vi "pregame.vi"() -> ()   [LabVIEW 2025]
uses:
  common/ClientNetworkInterfaceGlobalVariables.vi
  <vilib>/picture/picture.llb/Draw True-Color Pixmap.vi
panel:
  out "Game Field 2":picture
  out "Array 2":string[][](array[string])
  out "which type of box":i32
  out "team number":i32
  out "table of ID&team":i32[][](array[numeric])
  out "Table Control 3":string[][](table) caption="Table Control"
  out "seconds since 1Jan1904 3":timestamp
  out "speed":i32
  out "mountain_density":i32
  out "city_density":i32
  out "width":i32
  out "height":i32
  out "seconds since 1Jan1904 2":timestamp
  out "ACTION":T1
  out "seconds since 1Jan1904":timestamp
  out "map data 2":i32[][](array[numeric])
  in  "stop":bool
  in  "pen":T2={"Width"=1, "Style"=enum."Solid"}
  out "row":dbl
  out "col":dbl
  out "Numeric":i32
  in  "Array":string[][](array[string])
  out "Sent Message 7":string
  in  "Team":u8=1 max=15 step=1
  out "Sent Message 6":string
  out "Sent Message 5":string
  out "Sent Message 4":string
  out "Sent Message 3":string
  out "Sent Message":string
  out "Sent Message 2":string
  in  "Tab Control":enum32{"start", "PreGame", "InGame"}(tab)
  in  "exit":bool
  in  "play":bool
  out "Status":string
  in  "player_name":string
  in  "leave game":bool
  in  "PreGame menu":enum32{"Team", "Options"}(tab)
  in  "spectator":bool caption="Blank Button"
  in  "team5":bool caption="Blank Button"
  in  "team4":bool caption="Blank Button"
  in  "team3":bool caption="Blank Button"
  in  "team2":bool caption="Blank Button"
  in  "team1":bool caption="Blank Button"
  out "Table Control":string[][](table)
  in  "Speed":i32(slide) caption="Slide" scale=1.0..4.0
  in  "Map Width":i32(slide) caption="Slide" scale=10.0..20.0
  in  "Map Height":i32(slide) caption="Slide" scale=10.0..20.0
  in  "City Density":i32(slide) caption="Slide" scale=10.0..40.0
  in  "Mountain Density":i32(slide) caption="Slide" scale=10.0..60.0
  out "Status 2":string
  in  "Ready":bool
  in  "back_to _lobby":bool
  out "Turns":string
  in  "play 2":bool
  out "Game Field":picture
  out "Table Control 2":string[][](table) caption="Table Control"
  # "generals.io"
  # "generals.io"
  # "Protect your general. Capture enemy generals."
  # "Player Name¡G"
  # "Status"
  # "Status"
  # "select your team"
  # "Turn"
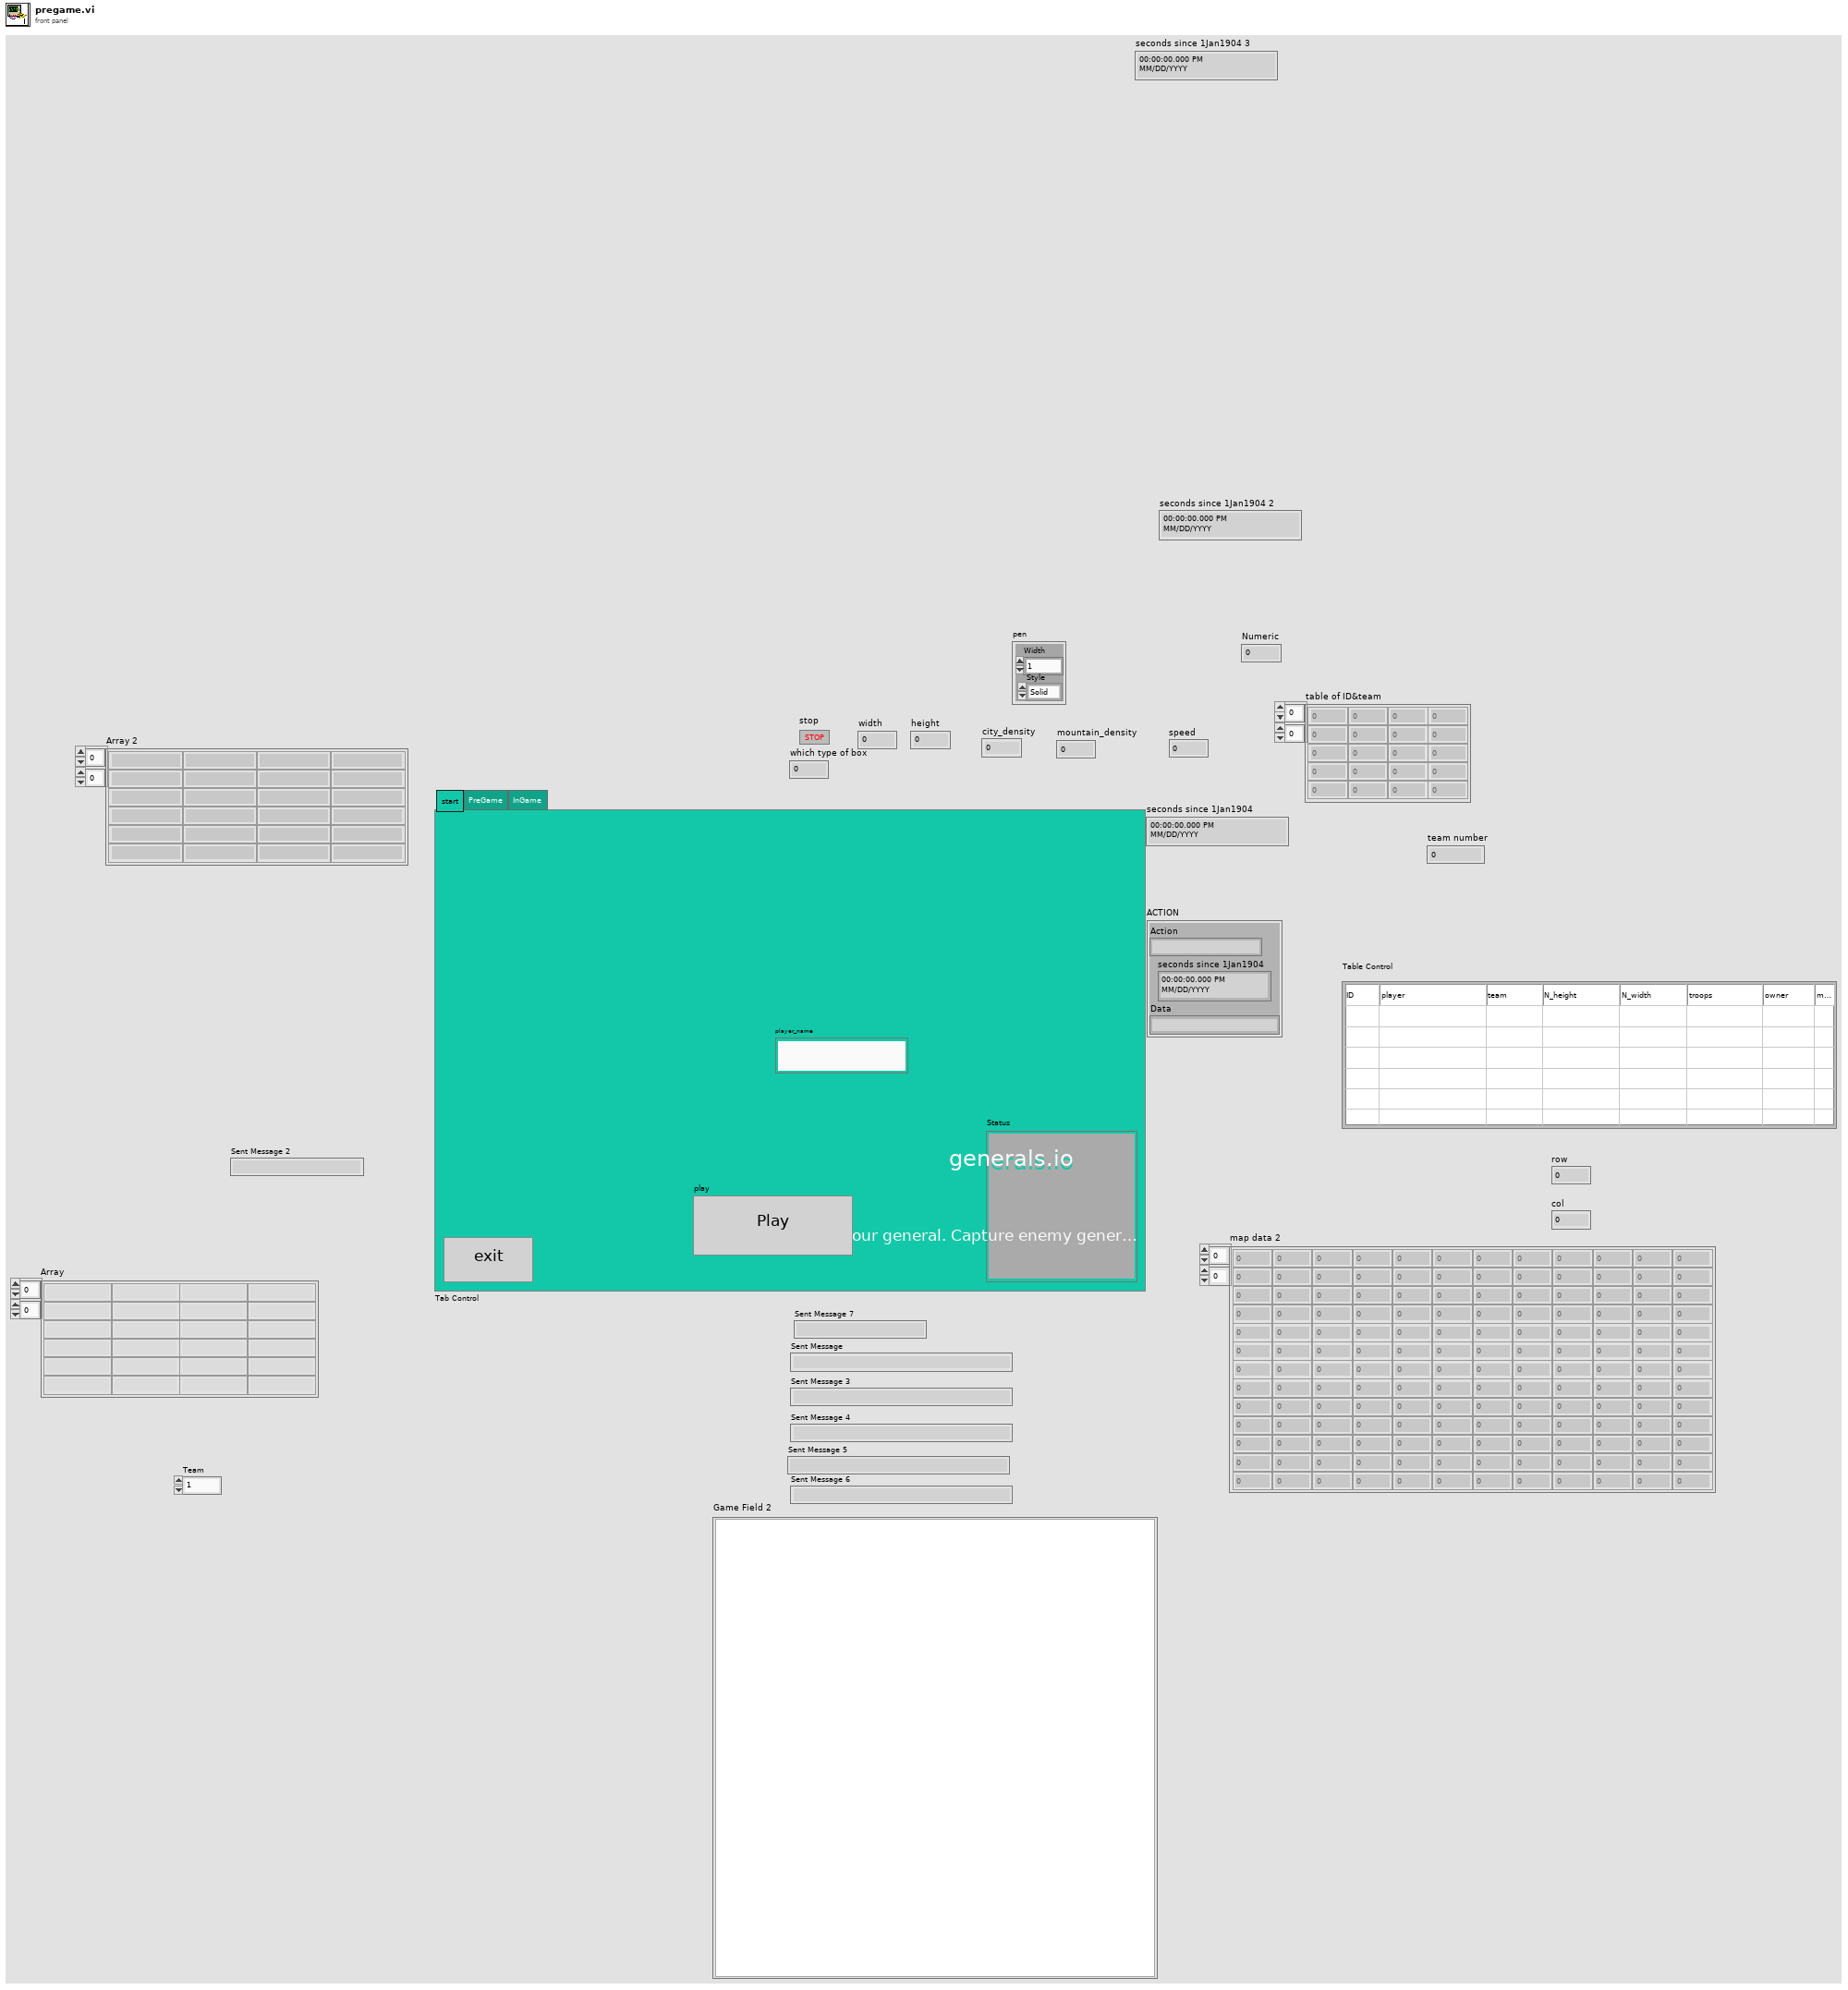
[diagram p1: front panel]
types:
  T1 = cluster{"Action":string, "seconds since 1Jan1904":timestamp, "Data":string}
  T2 = cluster{"Width":i16, "Style":enum32{"Solid", "Dash", "Dot", "DashDot", "DashDotDot"}}
  T3 = cluster{"seconds since 1Jan1904":timestamp, "Data":string}
  T4 = enum16{"Wait Send Queue Ready", "Wait Receive Queue Ready", "Poll Read Queue", "Process Data"}
  T5 = cluster{"Troops":u32, "Owner":i32, "Mountain":bool, "City":bool, "General":bool, "Fog":bool}[]
  T6 = map{u32, cluster{"Name":string, "Team":u8, "Ready":bool, "Host":bool, "Alive":bool, "Color":u32, "Lands":set{cluster{"Row":u32, "Column":u32}}, "Army":u32}}
  T7 = cluster{"Lands":set{cluster{"Row":u32, "Column":u32}}}[]
  T8 = typedef "imagedata.ctl" = cluster{"image type":i32, "image depth":i32, "image":u8[], "mask":u8[], "colors":u32[], "Rectangle":cluster{"left":i16, "top":i16, "right":i16, "bottom":i16}}
  T9 = typedef "LVPoint32TypeDef.ctl" = cluster{"Horizontal":i32, "Vertical":i32}
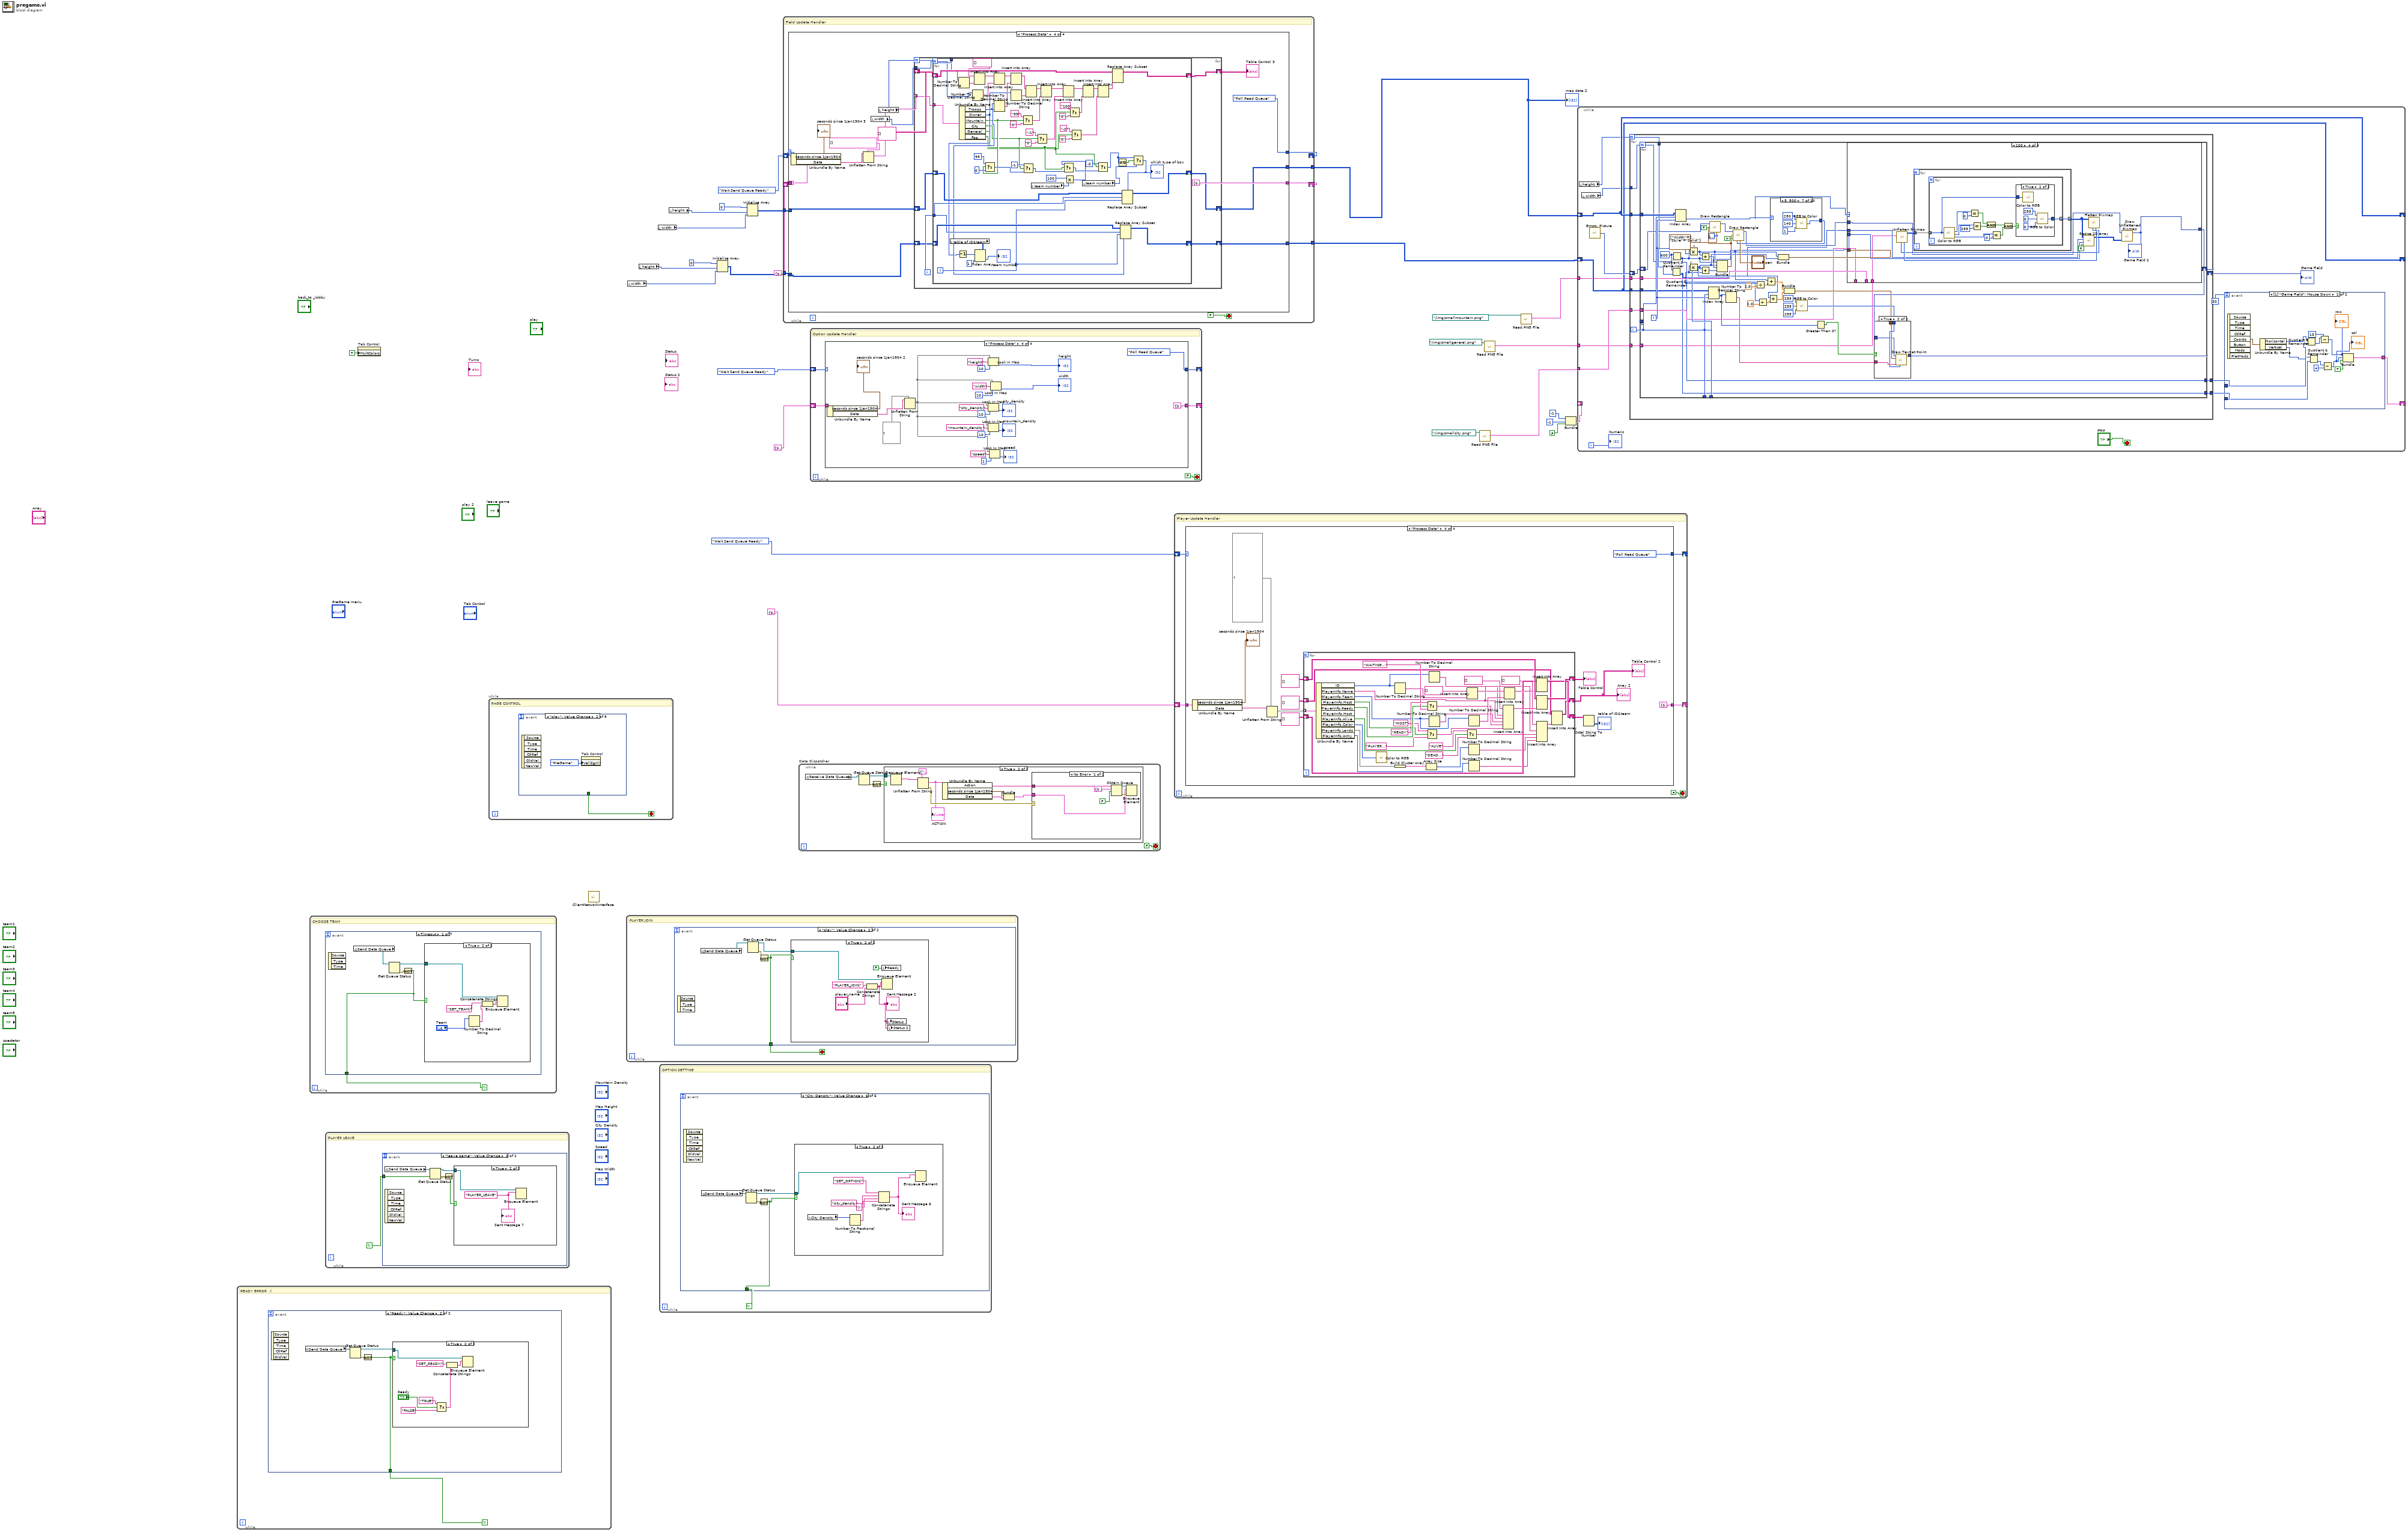
[diagram p0: block diagram]
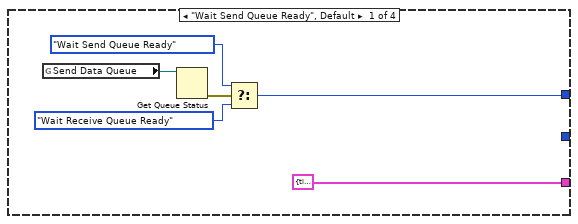
[diagram p2: hidden frame]
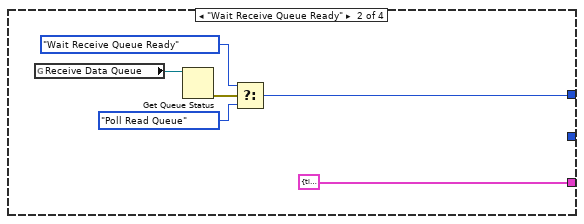
[diagram p3: hidden frame]
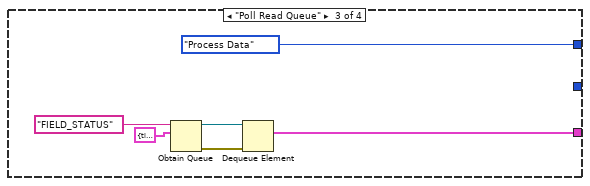
[diagram p4: hidden frame]
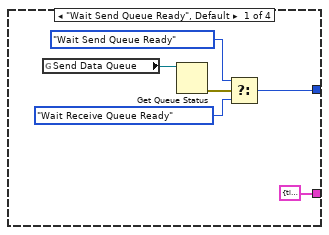
[diagram p5: hidden frame]
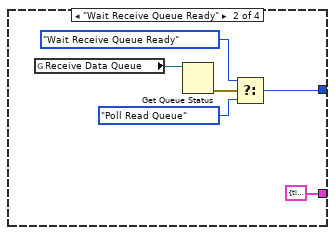
[diagram p6: hidden frame]
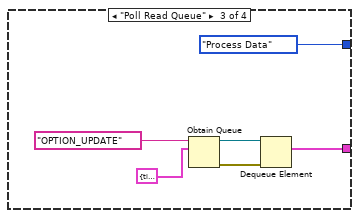
[diagram p7: hidden frame]
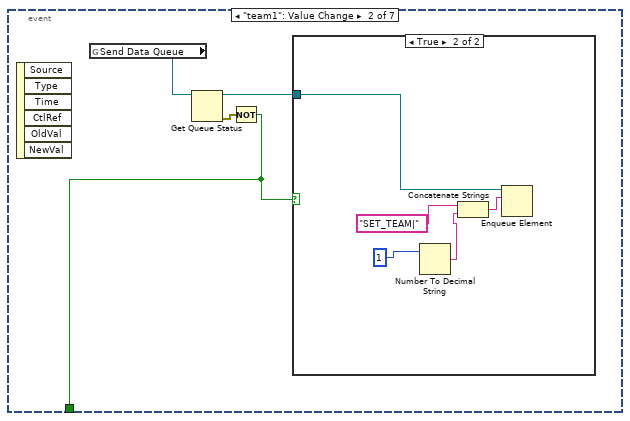
[diagram p9: hidden frame]
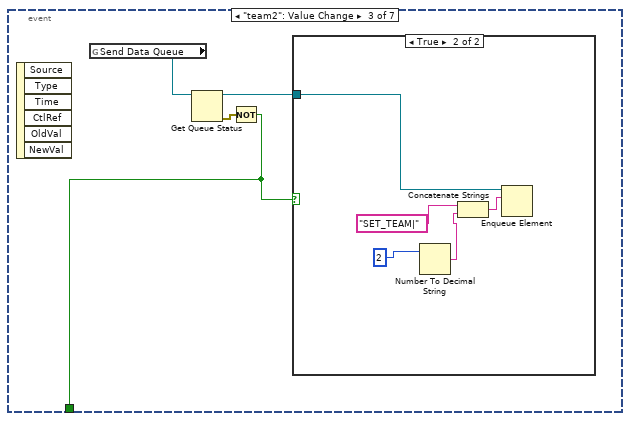
[diagram p11: hidden frame]
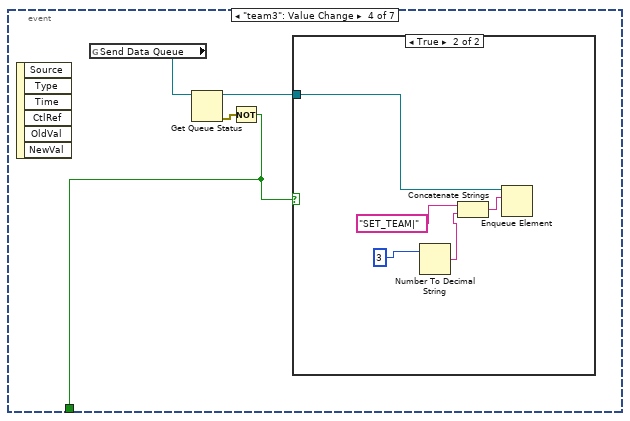
[diagram p13: hidden frame]
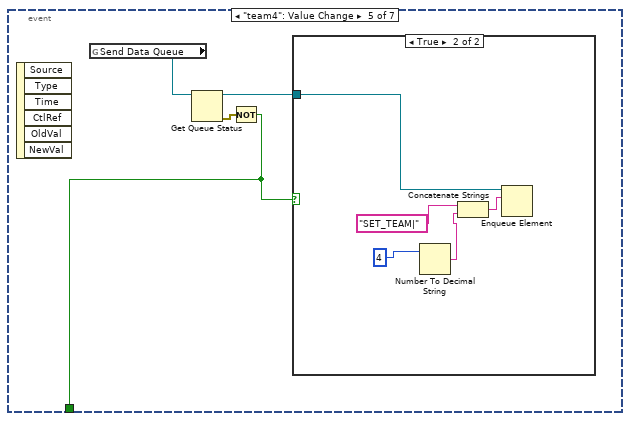
[diagram p15: hidden frame]
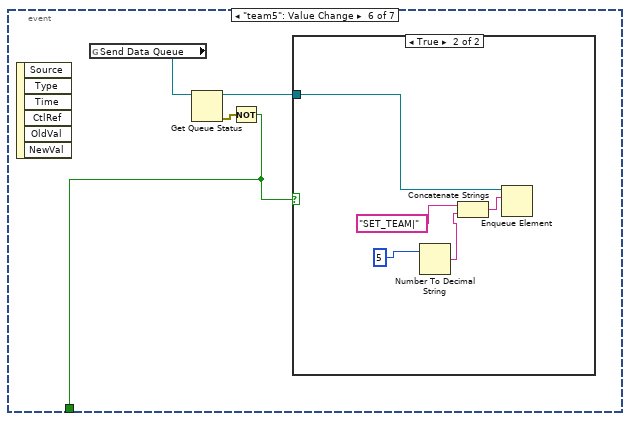
[diagram p17: hidden frame]
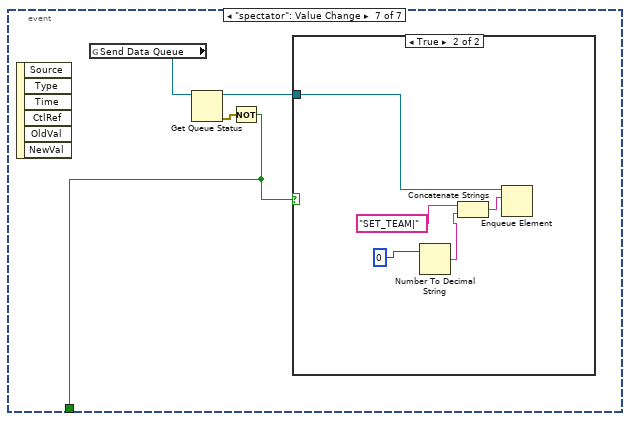
[diagram p19: hidden frame]
diagram:
  n1 = while {
    stop <- w28 continue-if-true
    # "READY ERROR  :("
    n2 = event shown="[1] \"Ready\": Value Change" {
      selector: _ -> [_ _]
      dyn-events: _ -> [_ _]
      timeout: _ -> [_ _]
      tunnel: [_ w29] -> w28
      event Timeout {
        n3 = event-data() -> ()  [unwired: 1 in, 3 out]
      }
      event "Ready": Value Change {
        n4 = event-data() -> ()  [unwired: 1 in, 5 out]
        n5 = global read "ClientNetworkInterfaceGlobalVariables.vi" "Send Data Queue"() -> (w32:refnum<queue>)
        n6 = Get Queue Status(queue=w32) -> (queue out=w31:refnum<queue>, error out=w30:errorcluster)  [unwired: 2 in, 6 out]
        n7 = Not(x=w30) -> (.not. x?=w29:bool)
        n8 = case shown="True" w29 {
          tunnel: w31 -> [_ w37]
          frame False {
          }
          frame True {
            n9 = Select(t="TRUE", s="Ready", f="FALSE") -> (s? t:f=w34:string)
            n10 = Concatenate Strings("SET_READY|" ("string"), w34) -> (w39:string)
            n11 = Enqueue Element(queue=w37, element=w39) -> ()  [unwired: 2 in, 3 out]
          }
        }
      }
    }
  }
  n12 = while {
    stop <- w40 continue-if-true
    # "CHOOSE TEAM"
    n13 = event shown="[0] Timeout" {
      selector: _ -> [_ _ _ _ _ _ _]
      dyn-events: _ -> [_ _ _ _ _ _ _]
      timeout: _ -> [_ _ _ _ _ _ _]
      tunnel: [w42 w51 w60 w69 w78 w87 w96] -> w40
      event Timeout {
        n14 = event-data() -> ()  [unwired: 1 in, 3 out]
        n15 = global read "ClientNetworkInterfaceGlobalVariables.vi" "Send Data Queue"() -> (w44:refnum<queue>)
        n16 = Get Queue Status(queue=w44) -> (queue out=w41:refnum<queue>, error out=w43:errorcluster)  [unwired: 2 in, 6 out]
        n17 = Not(x=w43) -> (.not. x?=w42:bool)
        n18 = case shown="True" w42 {
          tunnel: w41 -> [_ w46]
          frame False {
          }
          frame True {
            n19 = Number To Decimal String(number="Team") -> (decimal integer string=w47:string)  [unwired: 1 in]
            n20 = Concatenate Strings("SET_TEAM|" ("string"), w47) -> (w48:string)
            n21 = Enqueue Element(queue=w46, element=w48) -> ()  [unwired: 2 in, 3 out]
          }
        }
      }
      event "team1": Value Change {
        n22 = event-data() -> ()  [unwired: 1 in, 6 out]
        n23 = global read "ClientNetworkInterfaceGlobalVariables.vi" "Send Data Queue"() -> (w53:refnum<queue>)
        n24 = Get Queue Status(queue=w53) -> (queue out=w50:refnum<queue>, error out=w52:errorcluster)  [unwired: 2 in, 6 out]
        n25 = Not(x=w52) -> (.not. x?=w51:bool)
        n26 = case shown="True" w51 {
          tunnel: w50 -> [_ w55]
          frame False {
          }
          frame True {
            n27 = Number To Decimal String(number=1) -> (decimal integer string=w56:string)  [unwired: 1 in]
            n28 = Concatenate Strings("SET_TEAM|" ("string"), w56) -> (w57:string)
            n29 = Enqueue Element(queue=w55, element=w57) -> ()  [unwired: 2 in, 3 out]
          }
        }
      }
      event "team2": Value Change {
        n30 = event-data() -> ()  [unwired: 1 in, 6 out]
        n31 = global read "ClientNetworkInterfaceGlobalVariables.vi" "Send Data Queue"() -> (w62:refnum<queue>)
        n32 = Get Queue Status(queue=w62) -> (queue out=w59:refnum<queue>, error out=w61:errorcluster)  [unwired: 2 in, 6 out]
        n33 = Not(x=w61) -> (.not. x?=w60:bool)
        n34 = case shown="True" w60 {
          tunnel: w59 -> [_ w64]
          frame False {
          }
          frame True {
            n35 = Number To Decimal String(number=2) -> (decimal integer string=w65:string)  [unwired: 1 in]
            n36 = Concatenate Strings("SET_TEAM|" ("string"), w65) -> (w66:string)
            n37 = Enqueue Element(queue=w64, element=w66) -> ()  [unwired: 2 in, 3 out]
          }
        }
      }
      event "team3": Value Change {
        n38 = event-data() -> ()  [unwired: 1 in, 6 out]
        n39 = global read "ClientNetworkInterfaceGlobalVariables.vi" "Send Data Queue"() -> (w71:refnum<queue>)
        n40 = Get Queue Status(queue=w71) -> (queue out=w68:refnum<queue>, error out=w70:errorcluster)  [unwired: 2 in, 6 out]
        n41 = Not(x=w70) -> (.not. x?=w69:bool)
        n42 = case shown="True" w69 {
          tunnel: w68 -> [_ w73]
          frame False {
          }
          frame True {
            n43 = Number To Decimal String(number=3) -> (decimal integer string=w74:string)  [unwired: 1 in]
            n44 = Concatenate Strings("SET_TEAM|" ("string"), w74) -> (w75:string)
            n45 = Enqueue Element(queue=w73, element=w75) -> ()  [unwired: 2 in, 3 out]
          }
        }
      }
      event "team4": Value Change {
        n46 = event-data() -> ()  [unwired: 1 in, 6 out]
        n47 = global read "ClientNetworkInterfaceGlobalVariables.vi" "Send Data Queue"() -> (w80:refnum<queue>)
        n48 = Get Queue Status(queue=w80) -> (queue out=w77:refnum<queue>, error out=w79:errorcluster)  [unwired: 2 in, 6 out]
        n49 = Not(x=w79) -> (.not. x?=w78:bool)
        n50 = case shown="True" w78 {
          tunnel: w77 -> [_ w82]
          frame False {
          }
          frame True {
            n51 = Number To Decimal String(number=4) -> (decimal integer string=w83:string)  [unwired: 1 in]
            n52 = Concatenate Strings("SET_TEAM|" ("string"), w83) -> (w84:string)
            n53 = Enqueue Element(queue=w82, element=w84) -> ()  [unwired: 2 in, 3 out]
          }
        }
      }
      event "team5": Value Change {
        n54 = event-data() -> ()  [unwired: 1 in, 6 out]
        n55 = global read "ClientNetworkInterfaceGlobalVariables.vi" "Send Data Queue"() -> (w89:refnum<queue>)
        n56 = Get Queue Status(queue=w89) -> (queue out=w86:refnum<queue>, error out=w88:errorcluster)  [unwired: 2 in, 6 out]
        n57 = Not(x=w88) -> (.not. x?=w87:bool)
        n58 = case shown="True" w87 {
          tunnel: w86 -> [_ w91]
          frame False {
          }
          frame True {
            n59 = Number To Decimal String(number=5) -> (decimal integer string=w92:string)  [unwired: 1 in]
            n60 = Concatenate Strings("SET_TEAM|" ("string"), w92) -> (w93:string)
            n61 = Enqueue Element(queue=w91, element=w93) -> ()  [unwired: 2 in, 3 out]
          }
        }
      }
      event "spectator": Value Change {
        n62 = event-data() -> ()  [unwired: 1 in, 6 out]
        n63 = global read "ClientNetworkInterfaceGlobalVariables.vi" "Send Data Queue"() -> (w98:refnum<queue>)
        n64 = Get Queue Status(queue=w98) -> (queue out=w95:refnum<queue>, error out=w97:errorcluster)  [unwired: 2 in, 6 out]
        n65 = Not(x=w97) -> (.not. x?=w96:bool)
        n66 = case shown="True" w96 {
          tunnel: w95 -> [_ w100]
          frame False {
          }
          frame True {
            n67 = Number To Decimal String(number=0) -> (decimal integer string=w101:string)  [unwired: 1 in]
            n68 = Concatenate Strings("SET_TEAM|" ("string"), w101) -> (w102:string)
            n69 = Enqueue Element(queue=w100, element=w102) -> ()  [unwired: 2 in, 3 out]
          }
        }
      }
    }
  }
  n70 = while {
    stop <- w104 continue-if-true
    # "PLAYER LEAVE"
    n71 = event shown="[1] \"leave game\": Value Change" {
      selector: _ -> [_ _]
      dyn-events: _ -> [_ _]
      timeout: _ -> [_ _]
      tunnel: [_ w106] -> w104
      event Timeout {
        n72 = event-data() -> ()  [unwired: 1 in, 3 out]
      }
      event "leave game": Value Change {
        n73 = global read "ClientNetworkInterfaceGlobalVariables.vi" "Send Data Queue"() -> (w107:refnum<queue>)
        n74 = event-data() -> ()  [unwired: 1 in, 6 out]
        n75 = Get Queue Status(queue=w107) -> (queue out=w105:refnum<queue>, error out=w108:errorcluster)  [unwired: 2 in, 6 out]
        n76 = Not(x=w108) -> (.not. x?=w106:bool)
        n77 = case shown="True" w106 {
          tunnel: w105 -> [_ w109]
          frame False {
          }
          frame True {
            w110 = "PLAYER_LEAVE" ("string")
            n78 = Enqueue Element(queue=w109, element=w110) -> ()  [unwired: 2 in, 3 out]
            "Sent Message 7" <- w110
          }
        }
      }
    }
  }
  n79 = property on="Tab Control" class="TabCtl (strict)"("MultColors"=TRUE ("Allow Multiple Colors")) -> ()  [unwired: 2 in, 2 out]
  n80 = while {
    stop <- w111 stop-if-true
    # "PAGE CONTROL"
    n81 = event shown="[1] \"play\": Value Change" {
      selector: _ -> [_ _ _ _ _]
      dyn-events: _ -> [_ _ _ _ _]
      timeout: _ -> [_ _ _ _ _]
      tunnel: [_ _ _ _ "exit"] -> w111
      event Timeout {
        n82 = event-data() -> ()  [unwired: 1 in, 3 out]
      }
      event "play": Value Change {
        n83 = event-data() -> ()  [unwired: 1 in, 6 out]
        n84 = property on="Tab Control" class="TabCtl (strict)"("Val(Sgnl)"=enum32{"start", "PreGame", "InGame"}."PreGame" ("Value (Signaling)")) -> ()  [unwired: 2 in, 2 out]
      }
      event "leave game": Value Change {
        n85 = event-data() -> ()  [unwired: 1 in, 6 out]
        n86 = property on="Tab Control" class="TabCtl (strict)"("Val(Sgnl)"=enum32{"start", "PreGame", "InGame"}."start" ("Value (Signaling)")) -> ()  [unwired: 2 in, 2 out]
      }
      event "back_to _lobby": Value Change {
        n87 = event-data() -> ()  [unwired: 1 in, 6 out]
        n88 = property on="Tab Control" class="TabCtl (strict)"("Val(Sgnl)"=enum32{"start", "PreGame", "InGame"}."PreGame" ("Value (Signaling)")) -> ()  [unwired: 2 in, 2 out]
      }
      event "exit": Value Change {
        n89 = event-data() -> ()  [unwired: 1 in, 6 out]
      }
    }
  }
  n90 = call "ClientNetworkInterface.vi"() -> ()  [unwired: 1 in]
  n91 = while {
    stop <- w116 stop-if-true
    # "PLAYER JOIN"
    n92 = event shown="[1] \"play\": Value Change" {
      selector: _ -> [_ _]
      dyn-events: _ -> [_ _]
      timeout: _ -> [_ _]
      tunnel: [_ w117] -> w116
      event Timeout {
        n93 = event-data() -> ()  [unwired: 1 in, 3 out]
      }
      event "play": Value Change {
        n94 = event-data() -> ()  [unwired: 1 in, 3 out]
        n95 = global read "ClientNetworkInterfaceGlobalVariables.vi" "Send Data Queue"() -> (w118:refnum<queue>)
        n96 = Get Queue Status(queue=w118) -> (queue out=w119:refnum<queue>, error out=w120:errorcluster)  [unwired: 2 in, 6 out]
        n97 = Not(x=w120) -> (.not. x?=w117:bool)
        n98 = case shown="True" w117 {
          tunnel: w119 -> [_ w125]
          frame False {
          }
          frame True {
            n99 = Concatenate Strings("PLAYER_JOIN|" ("string"), "player_name") -> (w122:string)
            "Sent Message 2" <- w122
            n100 = local write "Ready"(FALSE ("Ready")) -> ()
            n101 = Enqueue Element(queue=w125, element=w122) -> ()  [unwired: 2 in, 3 out]
            n102 = local write "Status"(w122) -> ()
            n103 = local write "Status 2"(w122) -> ()
          }
        }
      }
    }
  }
  n104 = local read "width"() -> (w9:i32)
  n105 = local read "height"() -> (w8:i32)
  n106 = local read "width"() -> (w10:i32)
  n107 = while {
    stop <- w126 continue-if-true
    # "OPTION SETTING"
    n108 = event shown="[5] \"City Density\": Value Change" {
      selector: _ -> [_ _ _ _ _ _]
      dyn-events: _ -> [_ _ _ _ _ _]
      timeout: _ -> [_ _ _ _ _ _]
      tunnel: [_ w127 w139 w149 w160 w172] -> w126
      event Timeout {
        n109 = event-data() -> ()  [unwired: 1 in, 3 out]
      }
      event "Map Width": Value Change {
        n110 = event-data() -> ()  [unwired: 1 in, 6 out]
        n111 = global read "ClientNetworkInterfaceGlobalVariables.vi" "Send Data Queue"() -> (w129:refnum<queue>)
        n112 = Get Queue Status(queue=w129) -> (queue out=w128:refnum<queue>, error out=w130:errorcluster)  [unwired: 2 in, 6 out]
        n113 = Not(x=w130) -> (.not. x?=w127:bool)
        n114 = case shown="True" w127 {
          tunnel: w128 -> [_ w131]
          frame False {
          }
          frame True {
            n115 = local read "Map Width"() -> (w132:i32)
            n116 = Number To Fractional String(number=w132) -> (F-format string=w137:string)  [unwired: 3 in]
            n117 = Concatenate Strings("SET_OPTION|" ("string"), "width" ("Option"), "|" ("string"), w137) -> (w133:string)
            "Sent Message" <- w133
            n118 = Enqueue Element(queue=w131, element=w133) -> ()  [unwired: 2 in, 3 out]
          }
        }
      }
      event "Map Height": Value Change {
        n119 = event-data() -> ()  [unwired: 1 in, 6 out]
        n120 = global read "ClientNetworkInterfaceGlobalVariables.vi" "Send Data Queue"() -> (w140:refnum<queue>)
        n121 = Get Queue Status(queue=w140) -> (queue out=w138:refnum<queue>, error out=w141:errorcluster)  [unwired: 2 in, 6 out]
        n122 = Not(x=w141) -> (.not. x?=w139:bool)
        n123 = case shown="True" w139 {
          tunnel: w138 -> [_ w142]
          frame False {
          }
          frame True {
            n124 = local read "Map Height"() -> (w143:i32)
            n125 = Number To Fractional String(number=w143) -> (F-format string=w148:string)  [unwired: 3 in]
            n126 = Concatenate Strings("SET_OPTION|" ("string"), "height" ("Option"), "|" ("string"), w148) -> (w144:string)
            "Sent Message 3" <- w144
            n127 = Enqueue Element(queue=w142, element=w144) -> ()  [unwired: 2 in, 3 out]
          }
        }
      }
      event "Speed": Value Change {
        n128 = event-data() -> ()  [unwired: 1 in, 6 out]
        n129 = global read "ClientNetworkInterfaceGlobalVariables.vi" "Send Data Queue"() -> (w151:refnum<queue>)
        n130 = Get Queue Status(queue=w151) -> (queue out=w150:refnum<queue>, error out=w152:errorcluster)  [unwired: 2 in, 6 out]
        n131 = Not(x=w152) -> (.not. x?=w149:bool)
        n132 = case shown="True" w149 {
          tunnel: w150 -> [_ w153]
          frame False {
          }
          frame True {
            n133 = local read "Speed"() -> (w154:i32)
            n134 = Number To Fractional String(number=w154) -> (F-format string=w159:string)  [unwired: 3 in]
            n135 = Concatenate Strings("SET_OPTION|" ("string"), "speed" ("Option"), "|" ("string"), w159) -> (w155:string)
            "Sent Message 4" <- w155
            n136 = Enqueue Element(queue=w153, element=w155) -> ()  [unwired: 2 in, 3 out]
          }
        }
      }
      event "Mountain Density": Value Change {
        n137 = event-data() -> ()  [unwired: 1 in, 6 out]
        n138 = global read "ClientNetworkInterfaceGlobalVariables.vi" "Send Data Queue"() -> (w162:refnum<queue>)
        n139 = Get Queue Status(queue=w162) -> (queue out=w161:refnum<queue>, error out=w163:errorcluster)  [unwired: 2 in, 6 out]
        n140 = Not(x=w163) -> (.not. x?=w160:bool)
        n141 = case shown="True" w160 {
          tunnel: w161 -> [_ w164]
          frame False {
          }
          frame True {
            n142 = local read "Mountain Density"() -> (w165:i32)
            n143 = Number To Fractional String(number=w165) -> (F-format string=w170:string)  [unwired: 3 in]
            n144 = Concatenate Strings("SET_OPTION|" ("string"), "mountain_density" ("Option"), "|" ("string"), w170) -> (w166:string)
            "Sent Message 5" <- w166
            n145 = Enqueue Element(queue=w164, element=w166) -> ()  [unwired: 2 in, 3 out]
          }
        }
      }
      event "City Density": Value Change {
        n146 = event-data() -> ()  [unwired: 1 in, 6 out]
        n147 = global read "ClientNetworkInterfaceGlobalVariables.vi" "Send Data Queue"() -> (w173:refnum<queue>)
        n148 = Get Queue Status(queue=w173) -> (queue out=w171:refnum<queue>, error out=w174:errorcluster)  [unwired: 2 in, 6 out]
        n149 = Not(x=w174) -> (.not. x?=w172:bool)
        n150 = case shown="True" w172 {
          tunnel: w171 -> [_ w175]
          frame False {
          }
          frame True {
            n151 = local read "City Density"() -> (w176:i32)
            n152 = Number To Fractional String(number=w176) -> (F-format string=w181:string)  [unwired: 3 in]
            n153 = Concatenate Strings("SET_OPTION|" ("string"), "city_density" ("Option"), "|" ("string"), w181) -> (w177:string)
            "Sent Message 6" <- w177
            n154 = Enqueue Element(queue=w175, element=w177) -> ()  [unwired: 2 in, 3 out]
          }
        }
      }
    }
  }
  n155 = local read "height"() -> (w11:i32)
  n156 = Initialize Array(0, w8, w9) -> (w6:i32[][])
  n157 = Initialize Array(0, w11, w10) -> (w4:i32[][])
  n158 = while {
    shift-right: [w189] -> _
    shift-left: T4."Wait Send Queue Ready" -> [w186]
    shift-right: [w187] -> _
    shift-left: T3 {"seconds since 1Jan1904"=timestamp(0 s since 1904-01-01), "Data"=""} ("ActionDataCluster") -> [w188]
    tunnel: w6 -> [w185]
    tunnel: [w184] -> w5
    tunnel: w4 -> [w183]
    tunnel: [w182] -> w3
    stop <- FALSE stop-if-true
    # "Field Update Handler"
    n159 = case shown="\"Process Data\"" w186 {
      tunnel: [w195 w199 T4."Process Data" T4."Poll Read Queue"] -> w189
      tunnel: [T3 {"seconds since 1Jan1904"=timestamp(0 s since 1904-01-01), "Data"=""} ("ActionDataCluster") T3 {"seconds since 1Jan1904"=timestamp(0 s since 1904-01-01), "Data"=""} ("ActionDataCluster") w204 T3 {"seconds since 1Jan1904"=timestamp(0 s since 1904-01-01), "Data"=""} ("ActionDataCluster")] -> w187
      tunnel: w188 -> [_ _ _ w220]
      tunnel: w185 -> [_ _ _ w212]
      tunnel: [_ _ _ w211] -> w184
      tunnel: w183 -> [_ _ _ w210]
      tunnel: [_ _ _ w209] -> w182
      frame "Wait Send Queue Ready", Default {
        n160 = global read "ClientNetworkInterfaceGlobalVariables.vi" "Send Data Queue"() -> (w192:refnum<queue>)
        n161 = Get Queue Status(queue=w192) -> (error out=w196:errorcluster)  [unwired: 2 in, 7 out]
        n162 = Select(t=T4."Wait Send Queue Ready", s=w196, f=T4."Wait Receive Queue Ready") -> (s? t:f=w195:T4)
      }
      frame "Wait Receive Queue Ready" {
        n163 = global read "ClientNetworkInterfaceGlobalVariables.vi" "Receive Data Queue"() -> (w198:refnum<queue>)
        n164 = Get Queue Status(queue=w198) -> (error out=w202:errorcluster)  [unwired: 2 in, 7 out]
        n165 = Select(t=T4."Wait Receive Queue Ready", s=w202, f=T4."Poll Read Queue") -> (s? t:f=w199:T4)
      }
      frame "Poll Read Queue" {
        n166 = Obtain Queue(name (unnamed)="FIELD_STATUS", element data type=T3 {"seconds since 1Jan1904"=timestamp(0 s since 1904-01-01), "Data"=""} ("ActionDataCluster")) -> (queue out=w207:refnum<queue>, error out=w205:errorcluster)  [unwired: 3 in, 1 out]
        n167 = Dequeue Element(queue=w207, error in (no error)=w205) -> (element=w204:T3)  [unwired: 1 in, 3 out]
      }
      frame "Process Data" {
        n168 = Unbundle By Name(w220) -> ("seconds since 1Jan1904"=→"seconds since 1Jan1904 3":timestamp, "Data"=w219:string)
        n169 = Unflatten From String(type=T5 [] ("FieldArray"), binary string=w219) -> (value=w218:T5)  [unwired: 3 in, 2 out]
        n170 = local read "width"() -> (w214:i32)
        n171 = local read "height"() -> (w215:i32)
        n172 = for {
          N: w215 -> [w230]
          shift-right: [w231] -> w213
          shift-left: string[][] [] -> [w232]
          tunnel: w218 -> [w233] mode=indexing
          tunnel: w214 -> [w229]
          shift-right: [w226] -> w209
          shift-left: w210 -> [w227]
          shift-right: [w224] -> w211
          shift-left: w212 -> [w225]
          i -> [w228]
          n173 = for {
            N: w229 -> [w269]
            tunnel: w233 -> [w293]
            shift-right: [w291] -> w231
            shift-left: w232 -> [w292]
            tunnel: w230 -> [w268]
            tunnel: w228 -> [w258]
            shift-right: [w262] -> w226
            shift-left: w227 -> [w263]
            shift-right: [w260] -> w224
            shift-left: w225 -> [w261]
            i -> [w259]
            n174 = local read "table of ID&team"() -> (w256:i32[][])
            n175 = Number To Decimal String(number=w268) -> (decimal integer string=w274:string)  [unwired: 1 in]
            n176 = Unbundle By Name(w293) -> ("Troops"=w257:u32, "Owner"=w252:i32, "Mountain"=w244:bool, "City"=w243:bool, "General"=w242:bool, "Fog"=w241:bool)
            n177 = Decrement(x=w252) -> (x-1=w253:i32)
            n178 = Number To Decimal String(number=w269) -> (decimal integer string=w273:string)  [unwired: 1 in]
            n179 = Insert Into Array(array=string[] [], new element=w274) -> (w271:string[])  [unwired: 1 in]
            n180 = Index Array(array=w256, index (row)=w253, index (col)=1 ("disabled index (col)")) -> (element=→"team number":i32)
            n181 = Select(t=99, s=w244, f=0) -> (s? t:f=w248:i32)
            n182 = Insert Into Array(array=w271, new element=w273) -> (w270:string[])  [unwired: 1 in]
            n183 = Number To Decimal String(number=w257) -> (decimal integer string=w290:string)  [unwired: 1 in]
            n184 = Insert Into Array(array=w270, new element=w290) -> (w289:string[])  [unwired: 1 in]
            n185 = Number To Decimal String(number=w252) -> (decimal integer string=w288:string)  [unwired: 1 in]
            n186 = Select(t="99", s=w244, f="0") -> (s? t:f=w267:string)
            n187 = Select(t=-1, s=w243, f=w248) -> (s? t:f=w247:i32)
            n188 = Insert Into Array(array=w289, new element=w288) -> (w287:string[])  [unwired: 1 in]
            n189 = local read "team number"() -> (w240:i32)
            n190 = Select(t="-1", s=w243, f="0") -> (s? t:f=w266:string)
            n191 = Insert Into Array(array=w287, new element=w267) -> (w286:string[])  [unwired: 1 in]
            n192 = Insert Into Array(array=w286, new element=w266) -> (w285:string[])  [unwired: 1 in]
            n193 = Multiply(x=100 ("t"), y=w240) -> (x*y=w238:i32)
            n194 = Select(t=w238, s=w242, f=w247) -> (s? t:f=w245:i32)
            n195 = Select(t="100", s=w242, f="0") -> (s? t:f=w265:string)
            n196 = Select(t="-2", s=w241, f="0") -> (s? t:f=w264:string)
            n197 = local read "team number"() -> (w235:i32)
            n198 = Insert Into Array(array=w285, new element=w265) -> (w284:string[])  [unwired: 1 in]
            n199 = Select(t=-2, s=w241, f=w245) -> (s? t:f=w236:i32)
            n200 = Insert Into Array(array=w284, new element=w264) -> (w275:string[])  [unwired: 1 in]
            n201 = Replace Array Subset(array=w292, new element=w275) -> (w291:string[][])  [unwired: 2 in]
            n202 = Not Equal To 0?(x=w236) -> (x != 0?=w237:bool)
            n203 = Replace Array Subset(array=w261, new element=w257, index (row)=w258, index (col)=w259) -> (w260:i32[][])
            n204 = Select(t=w236, s=w237, f=w235) -> (s? t:f=w234:i32)
            "which type of box" <- w234
            n205 = Replace Array Subset(array=w263, new element=w234, index (row)=w258, index (col)=w259) -> (w262:i32[][])
          }
        }
        "Table Control 3" <- w213
      }
    }
  }
  "map data 2" <- w3
  n206 = while "Data Dispatcher" {
    stop <- FALSE stop-if-true
    n207 = global read "ClientNetworkInterfaceGlobalVariables.vi" "Receive Data Queue"() -> (w294:refnum<queue>)
    n208 = Get Queue Status(queue=w294) -> (queue out=w295:refnum<queue>, error out=w297:errorcluster)  [unwired: 2 in, 6 out]
    n209 = Not(x=w297) -> (.not. x?=w296:bool)
    n210 = case shown="True" w296 {
      tunnel: w295 -> [_ w307]
      frame False {
      }
      frame True {
        n211 = Dequeue Element(queue=w307) -> (element=w306:string)  [unwired: 2 in, 3 out]
        n212 = Unflatten From String(type=T1 {"Action"="", "seconds since 1Jan1904"=timestamp(0 s since 1904-01-01), "Data"=""} ("CommandCluster"), binary string=w306) -> (value=w299:T1, error out=w300:errorcluster)  [unwired: 3 in, 1 out]
        "ACTION" <- w299
        n213 = Unbundle By Name(w299) -> ("Action"=w301:string, "seconds since 1Jan1904"=w304:timestamp, "Data"=w303:string)
        n214 = Bundle("seconds since 1Jan1904"=w304, "Data"=w303) -> (w302:T3)  [unwired: 1 in]
        n215 = case shown="No Error" w300 {
          tunnel: w302 -> [w310 _]
          tunnel: w301 -> [w309 _]
          frame No Error {
            n216 = Obtain Queue(name (unnamed)=w309, element data type=T3 {"seconds since 1Jan1904"=timestamp(0 s since 1904-01-01), "Data"=""} ("ActionDataCluster"), create if not found? (T)=FALSE) -> (queue out=w312:refnum<queue>, error out=w311:errorcluster)  [unwired: 2 in, 1 out]
            n217 = Enqueue Element(queue=w312, element=w310, error in (no error)=w311) -> ()  [unwired: 1 in, 3 out]
          }
          frame Error {
          }
        }
      }
    }
  }
  n218 = while {
    shift-right: [w317] -> _
    shift-left: T4."Wait Send Queue Ready" -> [w314]
    shift-right: [w315] -> _
    shift-left: T3 {"seconds since 1Jan1904"=timestamp(0 s since 1904-01-01), "Data"=""} ("ActionDataCluster") -> [w316]
    stop <- FALSE stop-if-true
    # "Option Update Handler"
    n219 = case shown="\"Process Data\"" w314 {
      tunnel: [w323 w327 T4."Process Data" T4."Poll Read Queue"] -> w317
      tunnel: [T3 {"seconds since 1Jan1904"=timestamp(0 s since 1904-01-01), "Data"=""} ("ActionDataCluster") T3 {"seconds since 1Jan1904"=timestamp(0 s since 1904-01-01), "Data"=""} ("ActionDataCluster") w332 T3 {"seconds since 1Jan1904"=timestamp(0 s since 1904-01-01), "Data"=""} ("ActionDataCluster")] -> w315
      tunnel: w316 -> [_ _ _ w356]
      frame "Wait Send Queue Ready", Default {
        n220 = global read "ClientNetworkInterfaceGlobalVariables.vi" "Send Data Queue"() -> (w320:refnum<queue>)
        n221 = Get Queue Status(queue=w320) -> (error out=w324:errorcluster)  [unwired: 2 in, 7 out]
        n222 = Select(t=T4."Wait Send Queue Ready", s=w324, f=T4."Wait Receive Queue Ready") -> (s? t:f=w323:T4)
      }
      frame "Wait Receive Queue Ready" {
        n223 = global read "ClientNetworkInterfaceGlobalVariables.vi" "Receive Data Queue"() -> (w326:refnum<queue>)
        n224 = Get Queue Status(queue=w326) -> (error out=w330:errorcluster)  [unwired: 2 in, 7 out]
        n225 = Select(t=T4."Wait Receive Queue Ready", s=w330, f=T4."Poll Read Queue") -> (s? t:f=w327:T4)
      }
      frame "Poll Read Queue" {
        n226 = Obtain Queue(name (unnamed)="OPTION_UPDATE", element data type=T3 {"seconds since 1Jan1904"=timestamp(0 s since 1904-01-01), "Data"=""} ("ActionDataCluster")) -> (queue out=w335:refnum<queue>, error out=w333:errorcluster)  [unwired: 3 in, 1 out]
        n227 = Dequeue Element(queue=w335, error in (no error)=w333) -> (element=w332:T3)  [unwired: 1 in, 3 out]
      }
      frame "Process Data" {
        n228 = Unbundle By Name(w356) -> ("seconds since 1Jan1904"=→"seconds since 1Jan1904 2":timestamp, "Data"=w354:string)
        n229 = Unflatten From String(type=map{string, u32} {} ("Options"), binary string=w354) -> (value=w342:map{string, u32})  [unwired: 3 in, 2 out]
        n230 = Look In Map(map=w342, key="height", default value=u32 10) -> (value=→"height":u32)  [unwired: 1 out]
        n231 = Look In Map(map=w342, key="city_density", default value=u32 10) -> (value=→"city_density":u32)  [unwired: 1 out]
        n232 = Look In Map(map=w342, key="mountain_density", default value=u32 10) -> (value=→"mountain_density":u32)  [unwired: 1 out]
        n233 = Look In Map(map=w342, key="speed", default value=u32 1) -> (value=→"speed":u32)  [unwired: 1 out]
        n234 = Look In Map(map=w342, key="width", default value=u32 10) -> (value=→"width":u32)  [unwired: 1 out]
      }
    }
  }
  n235 = while {
    shift-right: [w362] -> _
    shift-left: T4."Wait Send Queue Ready" -> [w359]
    shift-right: [w360] -> _
    shift-left: T3 {"seconds since 1Jan1904"=timestamp(0 s since 1904-01-01), "Data"=""} ("ActionDataCluster") -> [w361]
    stop <- FALSE stop-if-true
    # "Player Update Handler"
    n236 = case shown="\"Process Data\"" w359 {
      tunnel: [w368 w372 T4."Process Data" T4."Poll Read Queue"] -> w362
      tunnel: [T3 {"seconds since 1Jan1904"=timestamp(0 s since 1904-01-01), "Data"=""} ("ActionDataCluster") T3 {"seconds since 1Jan1904"=timestamp(0 s since 1904-01-01), "Data"=""} ("ActionDataCluster") w377 T3 {"seconds since 1Jan1904"=timestamp(0 s since 1904-01-01), "Data"=""} ("ActionDataCluster")] -> w360
      tunnel: w361 -> [_ _ _ w391]
      frame "Wait Send Queue Ready", Default {
        n237 = global read "ClientNetworkInterfaceGlobalVariables.vi" "Send Data Queue"() -> (w365:refnum<queue>)
        n238 = Get Queue Status(queue=w365) -> (error out=w369:errorcluster)  [unwired: 2 in, 7 out]
        n239 = Select(t=T4."Wait Send Queue Ready", s=w369, f=T4."Wait Receive Queue Ready") -> (s? t:f=w368:T4)
      }
      frame "Wait Receive Queue Ready" {
        n240 = global read "ClientNetworkInterfaceGlobalVariables.vi" "Receive Data Queue"() -> (w371:refnum<queue>)
        n241 = Get Queue Status(queue=w371) -> (error out=w375:errorcluster)  [unwired: 2 in, 7 out]
        n242 = Select(t=T4."Wait Receive Queue Ready", s=w375, f=T4."Poll Read Queue") -> (s? t:f=w372:T4)
      }
      frame "Poll Read Queue" {
        n243 = Obtain Queue(name (unnamed)="PLAYER_UPDATE", element data type=T3 {"seconds since 1Jan1904"=timestamp(0 s since 1904-01-01), "Data"=""} ("ActionDataCluster")) -> (queue out=w380:refnum<queue>, error out=w378:errorcluster)  [unwired: 3 in, 1 out]
        n244 = Dequeue Element(queue=w380, error in (no error)=w378) -> (element=w377:T3)  [unwired: 1 in, 3 out]
      }
      frame "Process Data" {
        n245 = Unbundle By Name(w391) -> ("seconds since 1Jan1904"=→"seconds since 1Jan1904":timestamp, "Data"=w390:string)
        n246 = Unflatten From String(type=T6 {} ("PlayerInfoMap"), binary string=w390) -> (value=w389:T6)  [unwired: 3 in, 2 out]
        n247 = for {
          shift-right: [w433] -> w393
          shift-left: string[][] [] -> [w431]
          tunnel: w389 -> [w430] mode=indexing
          shift-right: [w421] -> w386
          shift-left: string[][] [] -> [w422]
          shift-right: [w413] -> w382
          shift-left: string[][] [] -> [w414]
          n248 = Unbundle By Name(w430) -> ("ID"=w418:u32, "PlayerInfo.Name"=w399:string, "PlayerInfo.Team"=w417:u8, "PlayerInfo.Host"=w426:bool, "PlayerInfo.Ready"=w429:bool, "PlayerInfo.Alive"=w410:bool, "PlayerInfo.Color"=w416:u32, "PlayerInfo.Lands"=w409:set{cluster{"Row":u32, "Column":u32}}, "PlayerInfo.Army"=w406:u32)  [unwired: 1 out]
          n249 = call <vilib>:"Color to RGB.vi"("Color"=w416) -> ()  [unwired: 4 out]
          n250 = Build Cluster Array(w409) -> (w408:T7)
          n251 = Number To Decimal String(number=w418) -> (decimal integer string=w419:string)  [unwired: 1 in]
          n252 = Array Size(array=w408) -> (size(s)=w407:i32)
          n253 = Select(t="READY", s=w429, f="WAITING...") -> (s? t:f=w401:string)
          n254 = Select(t="HOST", s=w426, f="PLAYER...") -> (s? t:f=w402:string)
          n255 = Number To Decimal String(number=w418) -> (decimal integer string=w398:string)  [unwired: 1 in]
          n256 = Number To Decimal String(number=w417) -> (decimal integer string=w400:string)  [unwired: 1 in]
          n257 = Select(t="ALIVE", s=w410, f="DEAD...") -> (s? t:f=w405:string)
          n258 = Insert Into Array(array=string[] [], new element=w419) -> (w424:string[])  [unwired: 1 in]
          n259 = Number To Decimal String(number=w417) -> (decimal integer string=w420:string)  [unwired: 1 in]
          n260 = Number To Decimal String(number=w407) -> (decimal integer string=w404:string)  [unwired: 1 in]
          n261 = Number To Decimal String(number=w406) -> (decimal integer string=w403:string)  [unwired: 1 in]
          n262 = Insert Into Array(array=string[] [], new element #1=w398, new element #2=w399, new element #3=w400, new element #4=w401, new element #5=w402) -> (w432:string[])  [unwired: 1 in]
          n263 = Insert Into Array(array=w424, new element=w420) -> (w423:string[])  [unwired: 1 in]
          n264 = Insert Into Array(array=w422, new element=w423) -> (w421:string[][])  [unwired: 2 in]
          n265 = Insert Into Array(array=w431, new element=w432) -> (w433:string[][])  [unwired: 2 in]
          n266 = Insert Into Array(array=string[] [], new element #1=w399, new element #2=w405, new element #3=w404, new element #4=w403) -> (w397:string[])  [unwired: 1 in]
          n267 = Insert Into Array(array=w414, new element=w397) -> (w413:string[][])  [unwired: 2 in]
        }
        "Table Control" <- w393
        "Array 2" <- w382
        "Table Control 2" <- w382
        n268 = Octal String To Number(4:w386) -> (0:→"table of ID&team":u32[][])  [unwired: 2 in, 1 out]
      }
    }
  }
  n269 = call <vilib>:"Read PNG File.vi"("path to PNG file"=path "../img/smallcity.png") -> ("image data"=w18:T8)  [unwired: 8 in, 2 out]
  n270 = call <vilib>:"Read PNG File.vi"("path to PNG file"=path "../img/smallgeneral.png") -> ("image data"=w1:T8)  [unwired: 8 in, 2 out]
  n271 = call <vilib>:"Read PNG File.vi"("path to PNG file"=path "../img/smallmountain.png") -> ("image data"=w24:T8)  [unwired: 8 in, 2 out]
  n272 = Bundle(-1, -1, FALSE) -> (w19:cluster{i32, i32, bool})  [unwired: 1 in]
  n273 = while {
    shift-right: [w447] -> _
    shift-left: w3 -> [w447]
    shift-right: [w446] -> _
    shift-left: w5 -> [w446]
    tunnel: w24 -> [w445]
    tunnel: w18 -> [w444]
    shift-right: [w441] -> _
    shift-left: w19 -> [_]
    tunnel: w1 -> [w436]
    i -> [w440]
    stop <- "stop" stop-if-true
    n274 = local read "height"() -> (w438:i32)
    n275 = local read "width"() -> (w437:i32)
    n276 = call "Empty Picture"() -> ("empty picture"=w448:picture)
    n277 = for {
      N: w438 -> [w473]
      shift-right: [w470] -> w449
      shift-left: w448 -> [w475]
      tunnel: w447 -> [w474]
      tunnel: w446 -> [w472]
      tunnel: w445 -> [w469]
      tunnel: w444 -> [w468]
      tunnel: [w467] -> w443
      tunnel: [w466] -> w442
      tunnel: w437 -> [w465]
      tunnel: w436 -> [w464]
      i -> [w471]
      n278 = for {
        N: w465 -> [w478]
        tunnel: w471 -> [w520]
        shift-right: [w496] -> w470
        shift-left: w475 -> [w494]
        tunnel: w474 -> [w516]
        tunnel: w473 -> [w479]
        tunnel: w471 -> [w515]
        tunnel: w472 -> [w513]
        tunnel: w471 -> [w512]
        tunnel: w469 -> [w487]
        tunnel: w468 -> [w482]
        tunnel: [w480] -> w467
        tunnel: [w481] -> w466
        tunnel: w464 -> [w477]
        i -> [w511]
        w521 = 600
        n279 = Quotient & Remainder(x=w521, y=w479) -> (floor(x/y)=w480:i32)  [unwired: 1 out]
        n280 = Quotient & Remainder(x=w521, y=w478) -> (floor(x/y)=w481:i32)  [unwired: 1 out]
        n281 = Index Array(array=w516, index (row)=w515, index (col)=w511) -> (element=w476:i32)
        n282 = Multiply "x"(x=w481, y=w511) -> (x*y=w485:i32)
        n283 = Multiply "y"(x=w480, y=w520) -> (x*y=w484:i32)
        n284 = Add(x=w485, y=w481) -> (x+y=w519:i32)
        n285 = Add(x=w484, y=w480) -> (x+y=w518:i32)
        n286 = Index Array(array=w513, index (row)=w512, index (col)=w511) -> (element=w500:i32)
        n287 = Bundle(w485, w484, w519, w518) -> (w486:cluster{i32, i32, i32, i32})  [unwired: 1 in]
        n288 = call <vilib>:"Draw Rectangle.vi"("picture"=w494, "rect"=w486, "fill?(F)"=FALSE, "color(black)"=u32 16777222, "pen"=T2 {"Width"=2, "Style"=enum."Solid"} ("pen 2")) -> ("new picture"=w493:picture)  [unwired: 4 in]
        n289 = Number To Decimal String(number=w500) -> (decimal integer string=w498:string)  [unwired: 1 in]
        n290 = Divide(x=w481, y=2.0) -> (x/y=w509:dbl)
        n291 = Divide(x=w480, y=2.0) -> (x/y=w508:dbl)
        n292 = Add(x=w485, y=w509) -> (x+y=w506:dbl)
        n293 = Add(x=w484, y=w508) -> (x+y=w505:dbl)
        n294 = case shown="5, 500" w476 {
          tunnel: [w576 w580 w584 w588 w592 w596 w600 w604 w608 w612] -> w514
          frame Default {
            n295 = call <vilib>:"RGB to Color.vi"("B"=255, "G"=255, "R"=255) -> ("Color"=w576:u32)
          }
          frame 0 {
            n296 = call <vilib>:"RGB to Color.vi"("B"=240, "G"=240, "R"=240) -> ("Color"=w580:u32)
          }
          frame 1, 100 {
            n297 = call <vilib>:"RGB to Color.vi"("B"=255, "G"=150, "R"=100) -> ("Color"=w584:u32)
          }
          frame 2, 200 {
            n298 = call <vilib>:"RGB to Color.vi"("B"=100, "G"=100, "R"=255) -> ("Color"=w588:u32)
          }
          frame 3, 300 {
            n299 = call <vilib>:"RGB to Color.vi"("B"=0, "G"=128, "R"=0) -> ("Color"=w592:u32)
          }
          frame 4, 400 {
            n300 = call <vilib>:"RGB to Color.vi"("B"=128, "G"=128, "R"=0) -> ("Color"=w596:u32)
          }
          frame 5, 500 {
            n301 = call <vilib>:"RGB to Color.vi"("B"=1, "G"=140, "R"=250) -> ("Color"=w600:u32)
          }
          frame 99 {
            n302 = call <vilib>:"RGB to Color.vi"("B"=80, "G"=80, "R"=80) -> ("Color"=w604:u32)
          }
          frame -1 {
            n303 = call <vilib>:"RGB to Color.vi"("B"=50, "G"=200, "R"=255) -> ("Color"=w608:u32)
          }
          frame -2 {
            n304 = call <vilib>:"RGB to Color.vi"("B"=0, "G"=0, "R"=0) -> ("Color"=w612:u32)
          }
        }
        n305 = call <vilib>:"Draw Rectangle.vi"("picture"=w493, "rect"=w486, "fill?(F)"=TRUE, "color(black)"=w514, "pen"="pen") -> ("new picture"=w489:picture)  [unwired: 4 in]
        n306 = Bundle(w485, w484) -> (w483:cluster{i32, i32})  [unwired: 1 in]
        n307 = Bundle(w506, w505) -> (w497:cluster{dbl, dbl})  [unwired: 1 in]
        n308 = call <vilib>:"RGB to Color.vi"("B"=255, "G"=255, "R"=255) -> ("Color"=w499:u32)
        n309 = Greater Than 0?(x=w500) -> (x > 0?=w501:bool)
        n310 = case shown="100" w476 {
          tunnel: w489 -> [w522 w529 w538 w542]
          tunnel: [w522 w527 w536 w543] -> w488
          tunnel: w487 -> [_ w530 _ _]
          tunnel: w483 -> [_ w528 w537 _]
          tunnel: w482 -> [_ _ w535 _]
          tunnel: w481 -> [_ w523 w532 w540]
          tunnel: w480 -> [_ w524 w531 w541]
          tunnel: w477 -> [_ _ _ w539]
          frame 0, Default {
          }
          frame 99 {
            n311 = call <vilib>:"Unflatten Pixmap.vi"("image data"=w530) -> ("24-bit pixmap"=w526:u32[][])  [unwired: 4 in, 6 out]
            n312 = call "Resize 2D array.vi"("New Width"=w523, "New Height"=w524, "2D Array In"=w526) -> ("Resized Array"=w525:u32[][])  [unwired: 4 in]
            n313 = call-poly <vilib>:"Draw Unflattened Pixmap.vi"("picture"=w529, "top left point(0, 0)"=w528, "data (RGB format)"=w525) -> ("new picture"=w527:picture)  [unwired: 6 in]
          }
          frame -1 {
            n314 = call <vilib>:"Unflatten Pixmap.vi"("image data"=w535) -> ("24-bit pixmap"=w534:u32[][])  [unwired: 4 in, 6 out]
            n315 = call "Resize 2D array.vi"("New Width"=w532, "New Height"=w531, "2D Array In"=w534) -> ("Resized Array"=w533:u32[][])  [unwired: 4 in]
            n316 = call-poly <vilib>:"Draw Unflattened Pixmap.vi"("picture"=w538, "top left point(0, 0)"=w537, "data (RGB format)"=w533) -> ("new picture"=w536:picture)  [unwired: 6 in]
          }
          frame 100 {
            n317 = call <vilib>:"Unflatten Pixmap.vi"("image data"=w539) -> ("24-bit pixmap"=w549:u32[][], "colors"=w547:u32[], "mask"=w544:u8[])  [unwired: 4 in, 4 out]
            n318 = for {
              tunnel: w549 -> [w551] mode=indexing
              tunnel: [w550] -> w548 mode=indexing
              n319 = for {
                tunnel: w551 -> [w552] mode=indexing
                tunnel: [w553] -> w550 mode=indexing
                n320 = call <vilib>:"Color to RGB.vi"("Color"=w552) -> ("R"=w564:u8, "G"=w560:u8, "B"=w559:u8)  [unwired: 1 out]
                n321 = Equal?(x=w564, y=u8 0) -> (x = y?=w558:bool)
                n322 = Equal?(x=w560, y=u8 255) -> (x = y?=w557:bool)
                n323 = And(x=w558, y=w557) -> (x .and. y?=w556:bool)
                n324 = Equal?(x=w559, y=u8 0) -> (x = y?=w555:bool)
                n325 = And(x=w556, y=w555) -> (x .and. y?=w554:bool)
                n326 = case shown="True" w554 {
                  tunnel: [_ w566] -> w553
                  tunnel: w552 -> [_ w565]
                  frame False {
                  }
                  frame True {
                    n327 = call <vilib>:"Color to RGB.vi"("Color"=w565) -> ()  [unwired: 4 out]
                    n328 = call <vilib>:"RGB to Color.vi"("B"=u8 0, "G"=u8 0, "R"=u8 255) -> ("Color"=w566:u32)
                  }
                }
              }
            }
            n329 = call "Resize 2D array.vi"("Maintain Aspect ratio? (T)"=FALSE, "New Width"=w540, "New Height"=w541, "2D Array In"=w548) -> ("Resized Array"=w545:u32[][])  [unwired: 3 in]
            n330 = call <vilib>:"Flatten Pixmap.vi"("mask"=w544, "colors"=w547, "24-bit pixmap"=w548) -> ()  [unwired: 8 in, 1 out]
            n331 = call-poly <vilib>:"Draw Unflattened Pixmap.vi"("picture"=w542, "data (RGB format)"=w545) -> ("new picture"=w543:picture)  [unwired: 7 in]
            "Game Field 2" <- w543
          }
        }
        n332 = case shown="True" w501 {
          tunnel: w499 -> [_ w575]
          tunnel: w498 -> [_ w574]
          tunnel: w497 -> [_ w573]
          tunnel: w488 -> [w570 w572]
          tunnel: [w570 w571] -> w496
          frame False {
          }
          frame True {
            n333 = call <vilib>:"Draw Text at Point.vi"("text color(black)"=w575, "text"=w574, "origin"=w573, "picture"=w572) -> ("new picture"=w571:picture)  [unwired: 6 in, 1 out]
          }
        }
      }
    }
    "Game Field" <- w449
    n334 = event shown="[1] \"Game Field\": Mouse Down" {
      selector: _ -> [_ _]
      dyn-events: _ -> [_ _]
      timeout: 30 -> [_ _]
      tunnel: w443 -> [_ w461]
      tunnel: w442 -> [_ w462]
      tunnel: [_ w459] -> w441
      event Timeout {
        n335 = event-data() -> ()  [unwired: 1 in, 3 out]
      }
      event "Game Field": Mouse Down {
        n336 = event-data() -> ("Coords"=w463:T9)  [unwired: 1 in, 7 out]
        n337 = Unbundle By Name(w463) -> ("Horizontal"=w458:i32, "Vertical"=w457:i32)
        n338 = Quotient & Remainder(x=w458, y=w462) -> (floor(x/y)=w455:i32)  [unwired: 1 out]
        n339 = Quotient & Remainder(x=w457, y=w461) -> (floor(x/y)=w453:i32)  [unwired: 1 out]
        n340 = Subtract(x=w455, y=13) -> (x-y=w456:i32)
        "row" <- w456
        n341 = Subtract(x=w453, y=4) -> (x-y=w452:i32)
        "col" <- w452
        n342 = Bundle(w456, w452, TRUE) -> (w459:cluster{i32, i32, bool})  [unwired: 1 in]
      }
    }
    "Numeric" <- w440
  }
